vi "MDPtr DecrementCount.vi"(9 "error in (no error)":errorcluster, 10 "HexStrPtr":T1) -> (2 "error out":errorcluster, 3 "HexStrPtr (dup)":T1)   [LabVIEW 2014]
uses:
  MDPtr TypeDef/MDPtr.ctl
  MDPtr TypeDef/MDPtr DataFrame-PlaceHolder.ctl
  MDPtr TypeDef/MDPtr DataFrame-Common.ctl
  MDPtr TypeDef/MDPtr SupportedDataTypeDef.ctl
  _Support/_MDPtr Build Error Cluster.vi
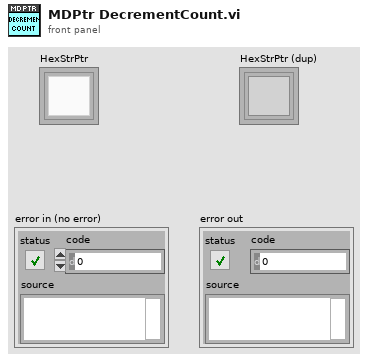
[diagram p1: front panel]
types:
  T1 = typedef "MDPtr.ctl" = refnum<k1>
  T2 = typedef "MDPtr DataFrame-PlaceHolder.ctl" = cluster{"Common":T3, "DVR":refnum<data-value>}
  T3 = typedef "MDPtr DataFrame-Common.ctl" = cluster{"Data Type":T4, "Copy Count":i32, "String Attribute":string}
  T4 = typedef "MDPtr SupportedDataTypeDef.ctl" = enum16{"<Invalid>", "Waveform", "Waveform Arr", "Double Arr", "String Arr"}
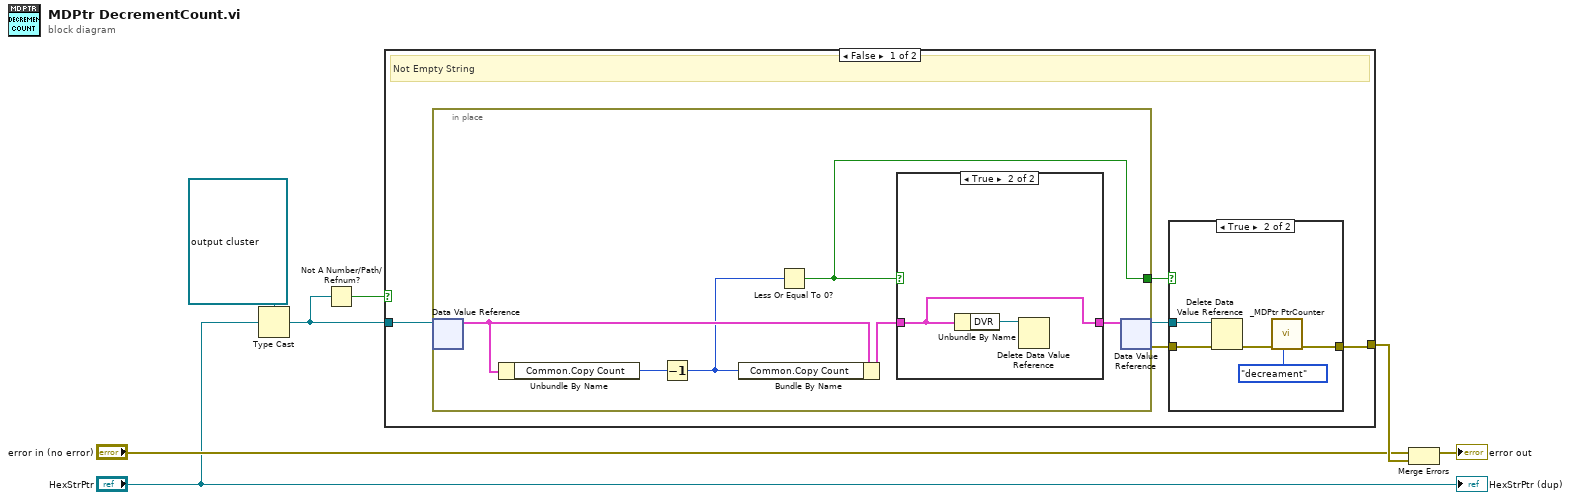
[diagram p0: block diagram]
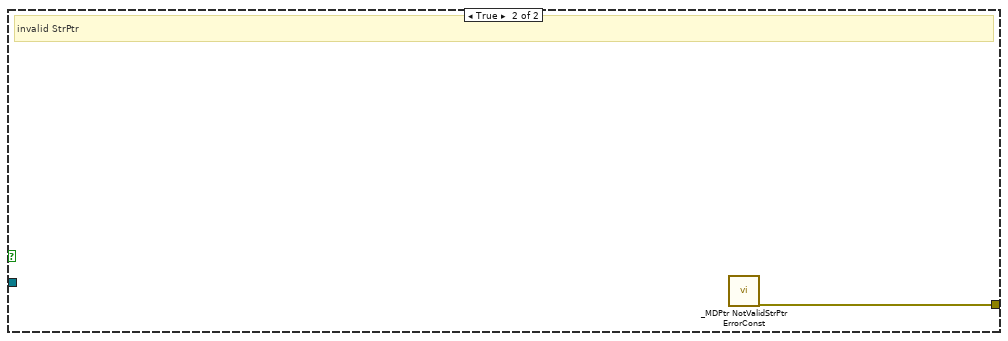
[diagram p4: hidden frame]
diagram:
  n1 = Type Cast(type=refnum<data-value> refnum ("data value reference"), x="HexStrPtr") -> (*(type *) &x=w1:refnum<data-value>)
  n2 = Not A Number/Path/Refnum?(number/path/refnum=w1) -> (NaN/Path/Refnum?=w2:bool)
  n3 = case shown="False" w2 {
    tunnel: [w10 w28] -> w7
    tunnel: w1 -> [w11 _]
    frame False {
      # "Not Empty String"
      n4 = in-place {
        in-place-border: [w22] -> w8
        n5 = in-place-dvr #1(w11) -> (w21:T2)  [unwired: 1 out]
        n6 = Unbundle By Name(w21) -> ("Common.Copy Count"=w20:i32)
        n7 = Decrement(x=w20) -> (x-1=w19:i32)
        n8 = Bundle By Name(cluster=w21, "Common.Copy Count"=w19) -> (w24:T2)
        n9 = Less Or Equal To 0?(x=w19) -> (x <= 0?=w22:bool)
        n10 = case shown="True" w22 {
          tunnel: w24 -> [w25 w26]
          tunnel: [w25 w26] -> w23
          frame False {
          }
          frame True {
            n11 = Unbundle By Name(w26) -> ("DVR"=w27:refnum<data-value>)
            n12 = Delete Data Value Reference(data value reference=w27) -> ()  [unwired: 1 in, 2 out]
          }
        }
        n13 = in-place-dvr #1(w23) -> (w9:refnum<data-value>, w12:errorcluster)
      }
      n14 = case shown="True" w8 {
        tunnel: w12 -> [w13 w18]
        tunnel: [w13 w15] -> w10
        tunnel: w9 -> [_ w16]
        frame False {
        }
        frame True {
          n15 = Delete Data Value Reference(data value reference=w16, error in=w18) -> (error out=w17:errorcluster)  [unwired: 1 out]
          n16 = call "_MDPtr PtrCounter.vi"("Oper(Get)"=enum16{"GET", "Increament", "decreament"}."decreament", "error in (no error)"=w17) -> ("error out"=w15:errorcluster)  [unwired: 8 in, 1 out]
        }
      }
    }
    frame True {
      # "invalid StrPtr"
      n17 = call "_MDPtr NotValidStrPtr ErrorConst.vi"() -> ("error out"=w28:errorcluster)  [unwired: 19 in]
    }
  }
  n18 = Merge Errors("error in (no error)", w7) -> (→"error out":errorcluster)
  "HexStrPtr (dup)" <- "HexStrPtr"
